vi "transition.vi"(8 "error in (no error)":errorcluster, 10 "Context In":refnum<class "Context.lvclass">, 11 "Stop in":refnum<class "Stop.lvclass">) -> (0 "error out":errorcluster, 2 "Context Out":refnum<class "Context.lvclass">, 3 "Stop out":refnum<class "Stop.lvclass">)   [LabVIEW 2018, in "Stop.lvclass"]
uses:
  Stop.lvclass
  Context/Context.lvclass
  Run/Run.lvclass
  C:/Users/fflores/Documents/OOP State Machine/State/State.lvclass
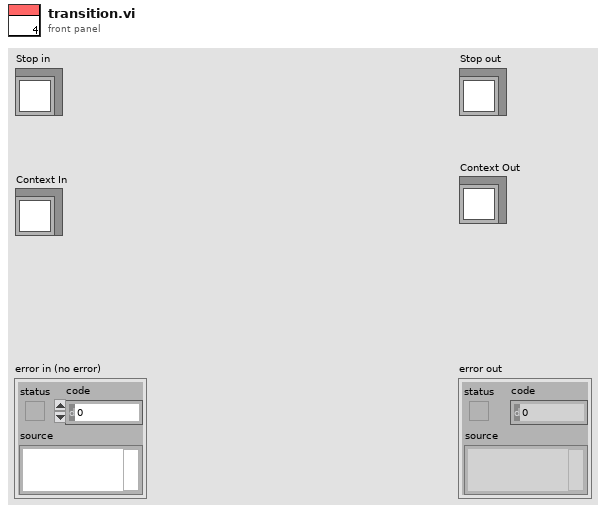
[diagram p1: front panel]
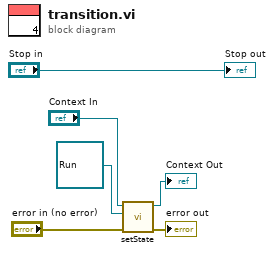
[diagram p0: block diagram]
diagram:
  n1 = call "setState.vi"("error in (no error)"="error in (no error)", "State.lvclass"=refnum<class "Run.lvclass"> refnum ("Run.lvclass"), "Context in"="Context In") -> ("error out"=→"error out":errorcluster, "Context out"=→"Context Out":refnum<class "Context.lvclass">)  [unwired: 7 in]
  "Stop out" <- "Stop in"
